vi "roi_setting_feedback.vi"(1 "input cluster":T2) -> (0 "output cluster":cluster{"destination":i16[][], dbl[]})   [LabVIEW 2010]
uses:
  <vilib>/vision/Image Controls.llb/IMAQ Image.ctl
  MWT_1.3.0_r1035/MultiWorm Tracker v1.3.0/data/MWT.dll
panel:
  out "size(s)":i32[](array[numeric])
  out "return type 2":i32
  out "return type":i32
  out "Image":T1(plugin-control)
  out "Numeric":i32
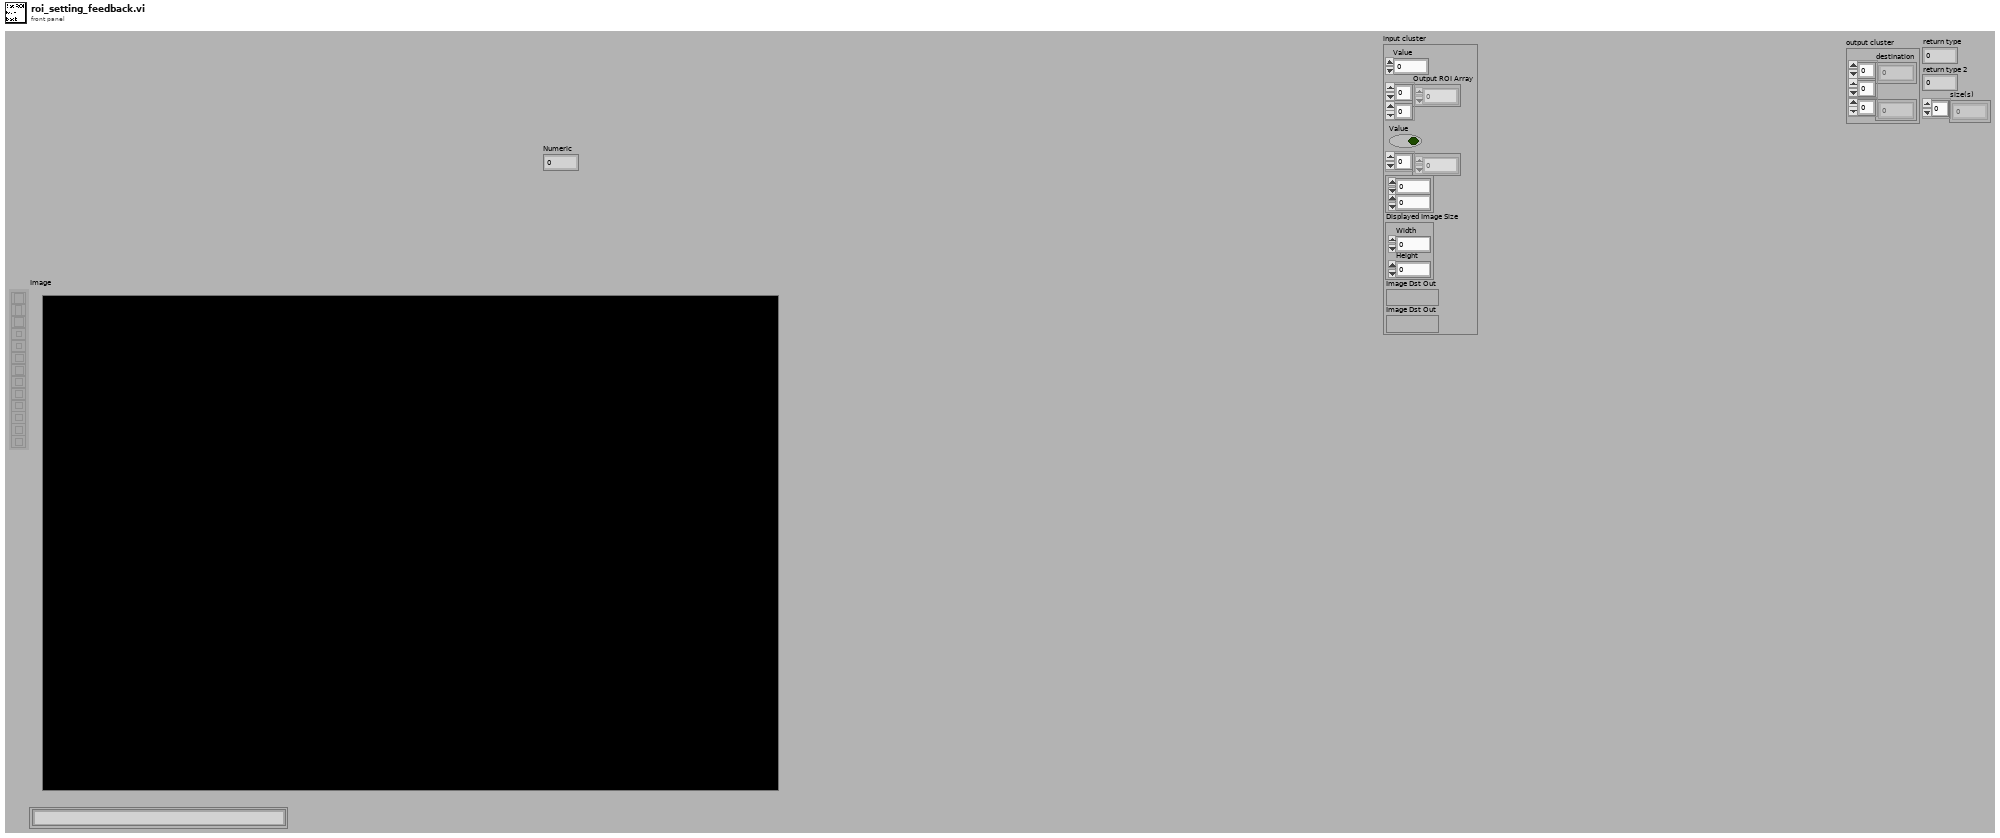
[diagram p1: front panel]
types:
  T1 = typedef "IMAQ Image.ctl" = refnum<image>
  T2 = cluster{"Value":i32, "Output ROI Array":dbl[][], "Value":bool, i32[], cluster{dbl, dbl}, "Displayed Image Size":cluster{"Width":u32, "Height":u32}, "Image Dst Out":T1, "Image Dst Out":T1}
  T3 = cluster{"[0]":i32, "[1]":i32, "[2]":i32, "[3]":i32}
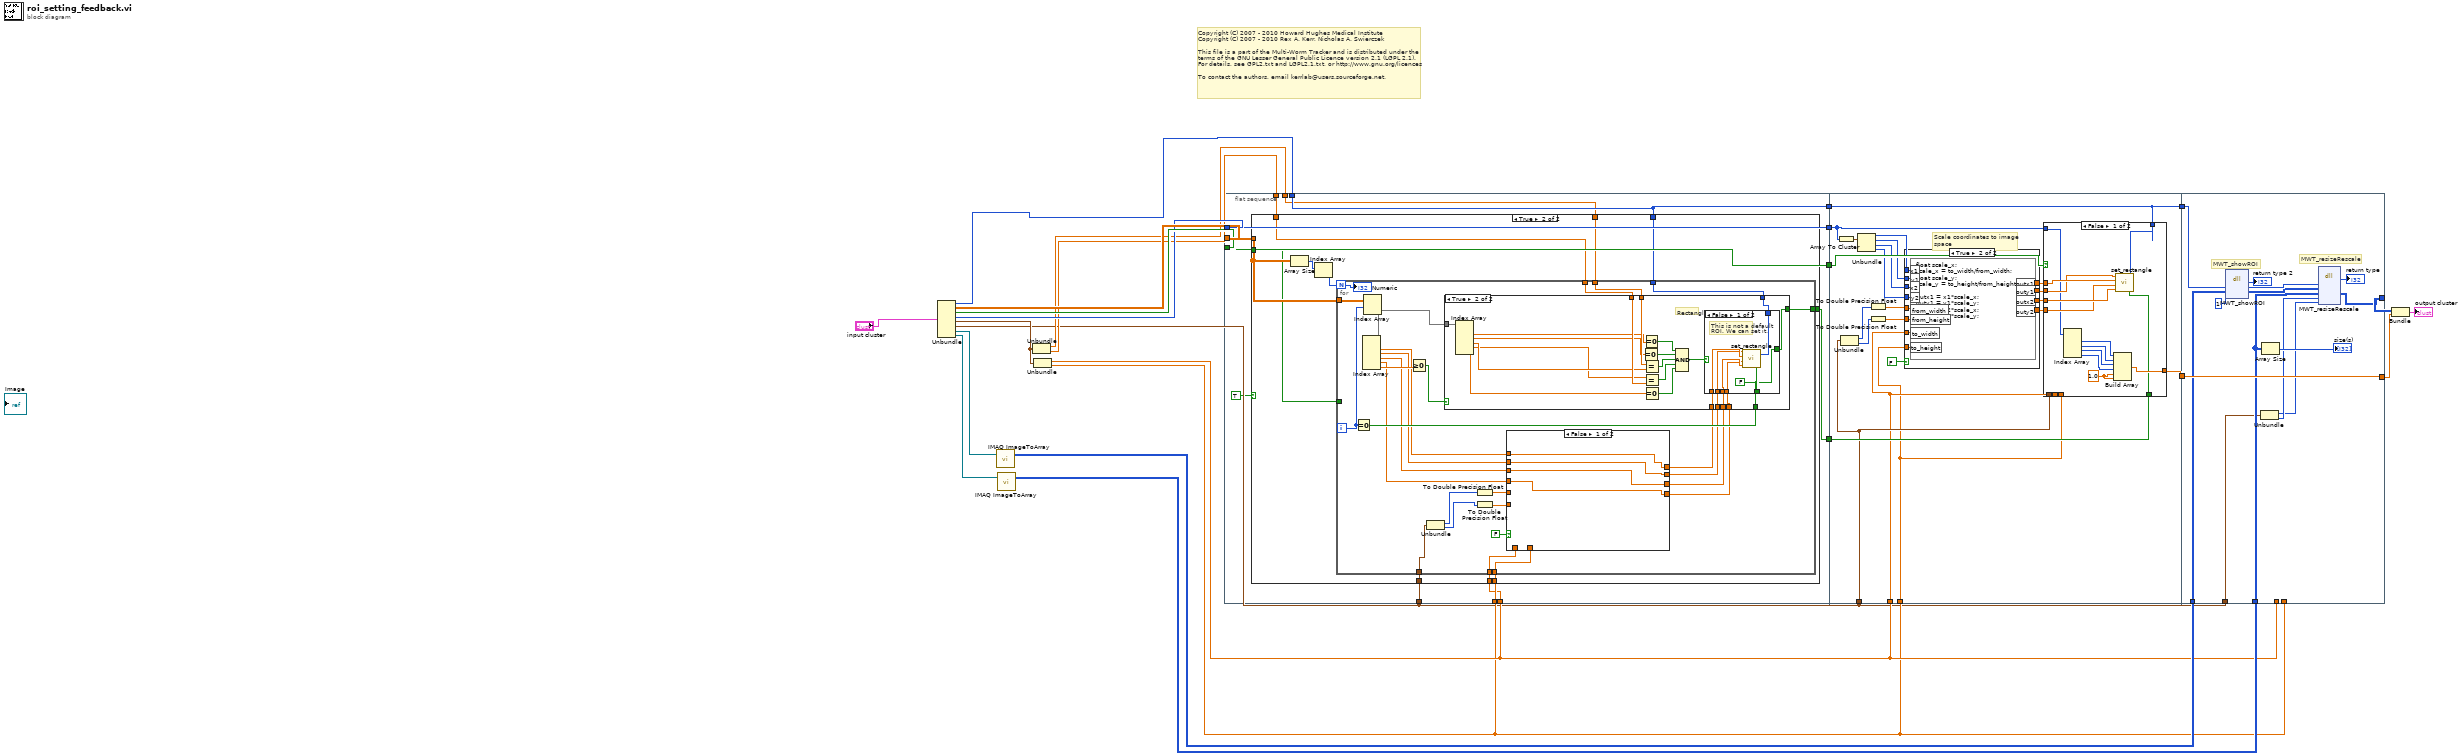
[diagram p0: block diagram]
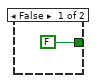
[diagram p2: hidden frame]
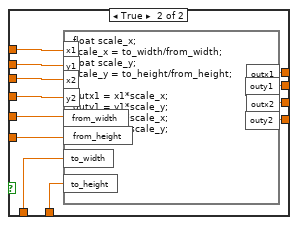
[diagram p3: hidden frame]
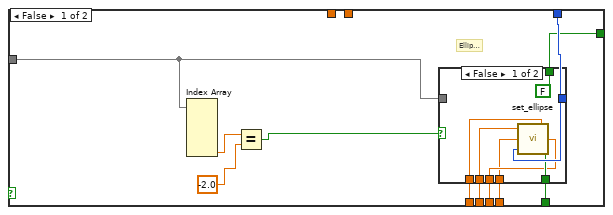
[diagram p4: hidden frame]
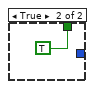
[diagram p5: hidden frame]
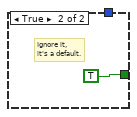
[diagram p6: hidden frame]
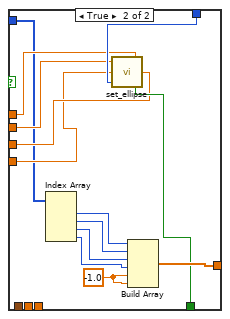
[diagram p8: hidden frame]
diagram:
  # "Copyright (C) 2007 - 2010 Howard Hughes Medical Institute\nCopyright (C) 2007 - 2010 Rex A. Kerr, Nicholas A. Swierczek\n \nThis file is a part of the Multi-Worm Tracker and is distributed under the\nterms of the GNU Lesser General Public Licence version 2.1 (LGPL 2.1).\nFor details, see GPL2.txt and LGPL2.1.txt, or http://www.gnu.org/licences\n \nTo contact the authors, email kerrlab@users.sourceforge.net."
  n1 = Unbundle("input cluster") -> ("Value"=w15:i32, "Output ROI Array"=w14:dbl[][], "Value"=w13:bool, w12:i32[], w4:cluster{dbl, dbl}, "Displayed Image Size"=w1:cluster{"Width":u32, "Height":u32}, "Image Dst Out"=w6:T1, "Image Dst Out"=w5:T1)
  n2 = call "IMAQ ImageToArray"("Image"=w6) -> ("Image Pixels (I16)"=w9:i16[][])  [unwired: 3 in, 4 out]
  n3 = call "IMAQ ImageToArray"("Image"=w5) -> ("Image Pixels (I16)"=w8:i16[][])  [unwired: 3 in, 4 out]
  n4 = Unbundle(w4) -> (w10:dbl, w11:dbl)
  n5 = Unbundle(w4) -> (w3:dbl, w2:dbl)
  n6 = flat-sequence {
    tunnel: w13 -> [w29]
    tunnel: w12 -> [w31]
    tunnel: w15 -> [w35]
    tunnel: [w35] -> w24
    tunnel: w14 -> [w34]
    tunnel: w10 -> [w33]
    tunnel: w11 -> [w32]
    tunnel: [w31] -> w23
    tunnel: [w29] -> w22
    tunnel: [w30] -> w21
    tunnel: w3 -> [w25]
    tunnel: w2 -> [w26]
    tunnel: w1 -> [w27]
    tunnel: w24 -> [w160]
    tunnel: [w160] -> w20
    tunnel: [w158] -> w19
    tunnel: w2 -> [w139]
    tunnel: w3 -> [w140]
    tunnel: w1 -> [w151]
    tunnel: w23 -> [w152]
    tunnel: w22 -> [w159]
    tunnel: w21 -> [w157]
    tunnel: w20 -> [w216]
    tunnel: w3 -> [_]
    tunnel: w2 -> [_]
    tunnel: w19 -> [w213]
    tunnel: w9 -> [w211]
    tunnel: w8 -> [w207]
    tunnel: [w206] -> w17
    tunnel: [w213] -> w18
    tunnel: w1 -> [w205]
    frame #0 {
      n7 = case shown="True" TRUE {
        tunnel: w35 -> [_ w47]
        tunnel: w34 -> [_ w46]
        tunnel: w33 -> [_ w43]
        tunnel: w32 -> [_ w42]
        tunnel: [FALSE w41] -> w30
        tunnel: w29 -> [_ w40]
        tunnel: w27 -> [_ w39]
        tunnel: w26 -> [_ w38]
        tunnel: w25 -> [_ w37]
        frame False {
        }
        frame True {
          n8 = Array Size(array=w46) -> (size(s)=w45:i32[])
          n9 = Index Array(array=w45) -> (element=w44:i32)  [unwired: 1 in]
          n10 = for {
            N: w44 -> [w70]
            tunnel: w46 -> [w72]
            tunnel: w47 -> [w74]
            tunnel: w43 -> [w68]
            tunnel: w42 -> [w67]
            tunnel: [w69] -> w41
            tunnel: w40 -> [_]
            tunnel: w39 -> [w53]
            tunnel: w38 -> [w50]
            tunnel: w37 -> [w49]
            i -> [w71]
            n11 = Equal To 0?(x=w71) -> (x = 0?=w73:bool)
            n12 = Index Array(array=w72, index (row)=w71) -> (element=w66:dbl[])  [unwired: 1 in]
            n13 = Index Array(array=w66) -> (element #1=w63:dbl, element #2=w62:dbl, element #3=w61:dbl, element #4=w60:dbl, element #5=w65:dbl)  [unwired: 5 in]
            n14 = Greater Or Equal To 0?(x=w65) -> (x >= 0?=w64:bool)
            n15 = Unbundle(w53) -> ("Width"=w54:u32, "Height"=w55:u32)
            n16 = To Double Precision Float(number=w54) -> (double precision float=w52:dbl)
            n17 = To Double Precision Float(number=w55) -> (double precision float=w51:dbl)
            n18 = case shown="False" FALSE {
              tunnel: w63 -> [w78 w90]
              tunnel: w62 -> [w77 w89]
              tunnel: w61 -> [w76 w88]
              tunnel: w60 -> [w75 w87]
              tunnel: [w78 w86] -> w59
              tunnel: [w77 w85] -> w58
              tunnel: [w76 w84] -> w57
              tunnel: [w75 w83] -> w56
              tunnel: w52 -> [_ w80]
              tunnel: w51 -> [_ w79]
              tunnel: w50 -> [_ w81]
              tunnel: w49 -> [_ w82]
              frame False {
              }
              frame True {
                n19 = formula code="float scale_x;\nscale_x = to_width/from_width;\nfloat scale_y;\nscale_y = to_height/from_height;\n\noutx1 = x1*scale_x;\nouty1 = y1*scale_y;\noutx2 = x2*scale_x;\nouty2 = y2*scale_y;"("x1"=w90, "y1"=w89, "x2"=w88, "y2"=w87, "from_width"=w80, "from_height"=w79, "to_width"=w82, "to_height"=w81) -> ("outx1"=w86:dbl, "outy1"=w85:dbl, "outx2"=w84:dbl, "outy2"=w83:dbl)
              }
            }
            n20 = case shown="True" w64 {
              tunnel: w66 -> [w98 w127]
              tunnel: w74 -> [w101 w130]
              tunnel: w73 -> [w100 w129]
              tunnel: [w99 w128] -> w69
              tunnel: w68 -> [_ w126]
              tunnel: w67 -> [_ w125]
              tunnel: w59 -> [w94 w113]
              tunnel: w58 -> [w93 w112]
              tunnel: w57 -> [w92 w111]
              tunnel: w56 -> [w91 w110]
              frame False {
                # "Ellipse"
                n21 = Index Array(array=w98) -> (element #5=w97:dbl)  [unwired: 5 in, 4 out]
                n22 = Equal?(x=w97, y=-2.0) -> (x = y?=w95:bool)
                n23 = case shown="False" w95 {
                  tunnel: w98 -> [_ _]
                  tunnel: w101 -> [w108 _]
                  tunnel: w100 -> [w107 _]
                  tunnel: [FALSE TRUE] -> w99
                  tunnel: w94 -> [w105 _]
                  tunnel: w93 -> [w104 _]
                  tunnel: w92 -> [w103 _]
                  tunnel: w91 -> [w102 _]
                  frame False {
                    n24 = call "set_ellipse.vi"("Set/Add"=w107, "y2"=w103, "y1"=w105, "Handle"=w108, "x2"=w102, "x1"=w104) -> ()
                  }
                  frame True {
                  }
                }
              }
              frame True {
                # "Rectangle"
                n25 = Index Array(array=w127) -> (element #1=w117:dbl, element #2=w116:dbl, element #3=w115:dbl, element #4=w114:dbl, element #5=w119:dbl)  [unwired: 5 in]
                n26 = Equal To 0?(x=w116) -> (x = 0?=w123:bool)
                n27 = Equal To 0?(x=w117) -> (x = 0?=w124:bool)
                n28 = Equal?(x=w126, y=w115) -> (x = y?=w122:bool)
                n29 = Equal?(x=w114, y=w125) -> (x = y?=w121:bool)
                n30 = Equal To 0?(x=w119) -> (x = 0?=w118:bool)
                n31 = Compound Arithmetic op=AND(w124, w123, w122, w121, w118) -> (w120:bool)
                n32 = case shown="False" w120 {
                  tunnel: w130 -> [w137 _]
                  tunnel: w129 -> [w136 _]
                  tunnel: [FALSE TRUE] -> w128
                  tunnel: w113 -> [w134 _]
                  tunnel: w112 -> [w133 _]
                  tunnel: w111 -> [w132 _]
                  tunnel: w110 -> [w131 _]
                  frame False {
                    # "This is not a default\nROI. We can set it."
                    n33 = call "set_rectangle.vi"("Set/Add"=w136, "Handle"=w137, "y2"=w132, "x2"=w131, "y1"=w134, "x1"=w133) -> ()
                  }
                  frame True {
                    # "Ignore it,\nit's a default."
                  }
                }
              }
            }
            "Numeric" <- w70
          }
        }
      }
    }
    frame #1 {
      # "Scale coordinates to image\nspace"
      n34 = Array To Cluster(array=w152) -> (cluster=w156:T3)
      n35 = Unbundle(w151) -> ("Width"=w145:u32, "Height"=w144:u32)
      n36 = Unbundle(w156) -> ("[0]"=w150:i32, "[1]"=w155:i32, "[2]"=w154:i32, "[3]"=w153:i32)
      n37 = To Double Precision Float(number=w145) -> (double precision float=w142:dbl)
      n38 = To Double Precision Float(number=w144) -> (double precision float=w141:dbl)
      n39 = case shown="True" FALSE {
        tunnel: w142 -> [_ w176]
        tunnel: w155 -> [w163 w175]
        tunnel: w154 -> [w162 w174]
        tunnel: w153 -> [w161 w173]
        tunnel: w150 -> [w164 w172]
        tunnel: [w164 w171] -> w149
        tunnel: [w163 w170] -> w148
        tunnel: [w162 w169] -> w147
        tunnel: [w161 w168] -> w146
        tunnel: w141 -> [_ w167]
        tunnel: w140 -> [_ w166]
        tunnel: w139 -> [_ w165]
        frame False {
        }
        frame True {
          n40 = formula code="float scale_x;\nscale_x = to_width/from_width;\nfloat scale_y;\nscale_y = to_height/from_height;\n\noutx1 = x1*scale_x;\nouty1 = y1*scale_y;\noutx2 = x2*scale_x;\nouty2 = y2*scale_y;"("x1"=w172, "y1"=w175, "x2"=w174, "y2"=w173, "from_width"=w176, "from_height"=w167, "to_width"=w166, "to_height"=w165) -> ("outx1"=w171:dbl, "outy1"=w170:dbl, "outx2"=w169:dbl, "outy2"=w168:dbl)
        }
      }
      n41 = case shown="False" w159 {
        tunnel: w152 -> [w181 w194]
        tunnel: w160 -> [w189 w202]
        tunnel: w140 -> [_ _]
        tunnel: w139 -> [_ _]
        tunnel: w151 -> [_ _]
        tunnel: [w188 w201] -> w158
        tunnel: w157 -> [w187 w200]
        tunnel: w149 -> [w185 w198]
        tunnel: w148 -> [w184 w195]
        tunnel: w147 -> [w183 w197]
        tunnel: w146 -> [w182 w196]
        frame False {
          w186 = 1.0 ("element")
          n42 = Index Array(array=w181) -> (element #1=w180:i32, element #2=w179:i32, element #3=w178:i32, element #4=w177:i32)  [unwired: 4 in]
          n43 = Build Array(w180, w179, w178, w177, w186, w186) -> (w188:dbl[])
          n44 = call "set_rectangle.vi"("Set/Add"=w187, "Handle"=w189, "y2"=w183, "x2"=w182, "y1"=w185, "x1"=w184) -> ()
        }
        frame True {
          w199 = -1.0 ("element")
          n45 = Index Array(array=w194) -> (element #1=w193:i32, element #2=w192:i32, element #3=w191:i32, element #4=w190:i32)  [unwired: 4 in]
          n46 = call "set_ellipse.vi"("Set/Add"=w200, "y2"=w197, "y1"=w198, "Handle"=w202, "x2"=w196, "x1"=w195) -> ()
          n47 = Build Array(w193, w192, w191, w190, w199, w199) -> (w201:dbl[])
        }
      }
    }
    frame #2 {
      # "MWT_resizeRescale"
      # "MWT_showROI"
      n48 = dll-call lib="C:/Users/Marc/multi worm tracker/MWT_1.3.0_r1035/MultiWorm Tracker v1.3.0/data/MWT.dll" fn="MWT_showROI"("handle"=w216, "image"=w211, "bin"=1) -> ("return type"=→"return type 2":i32, "handle"=w215:i32, "image"=w214:i16[][])  [unwired: 4 in, 2 out]
      n49 = Unbundle(w205) -> ("Width"=w203:u32, "Height"=w204:u32)
      n50 = Array Size(array=w207) -> (size(s)=→"size(s)":i32[])
      n51 = dll-call lib="C:/Users/Marc/multi worm tracker/MWT_1.3.0_r1035/MultiWorm Tracker v1.3.0/data/MWT.dll" fn="MWT_resizeRescale"("handle"=w215, "source"=w214, "destination"=w207, "width"=w204, "height"=w203) -> ("return type"=→"return type":i32, "destination"=w206:i16[][])  [unwired: 7 in, 2 out]
    }
  }
  n52 = Bundle("destination"=w17, w18) -> (→"output cluster":cluster{"destination":i16[][], dbl[]})  [unwired: 1 in]
